vi "Destroy.vi"(8 "error in (no error)":errorcluster, 11 "Event Registration Refnum":refnum<event-registration>) -> (0 "error out":errorcluster)   [LabVIEW 2020, in "WebServiceImporter.lvlib" / "Main Panel.lvlib" / "Input WSDL.lvlib" / "Events.lvlib"]
uses:
  <vilib>/Platform/WebService/Main Panel/Pages/Input WSDL/Events/Events.lvlib
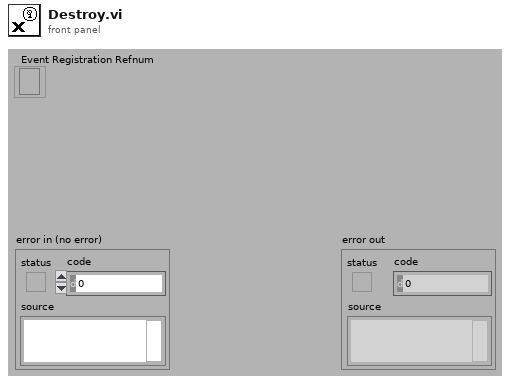
[diagram p1: front panel]
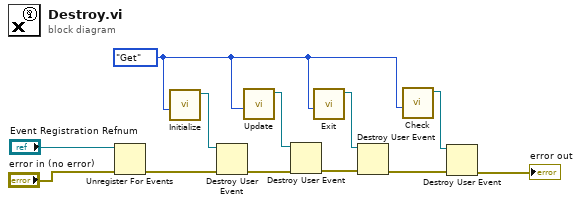
[diagram p0: block diagram]
diagram:
  w1 = enum16{"Get", "Set"}."Get" ("Operation")
  n1 = Unregister For Events(event registration refnum="Event Registration Refnum", error in="error in (no error)") -> (error out=w11:errorcluster)
  n2 = call <vilib>:"Initialize.vi"("Operation"=w1) -> ("user event (out)"=w10:refnum<user-event>)  [unwired: 10 in]
  n3 = Destroy User Event(user event=w10, error in=w11) -> (error out=w4:errorcluster)
  n4 = call <vilib>:"Update.vi"("Operation"=w1) -> ("user event (out)"=w2:refnum<user-event>)  [unwired: 9 in, 1 out]
  n5 = Destroy User Event(user event=w2, error in=w4) -> (error out=w3:errorcluster)
  n6 = call <vilib>:"Exit.vi"("Operation"=w1) -> ("user event (out)"=w9:refnum<user-event>)  [unwired: 9 in, 1 out]
  n7 = Destroy User Event(user event=w9, error in=w3) -> (error out=w8:errorcluster)
  n8 = call <vilib>:"Check.vi"("Operation"=w1) -> ("user event (out)"=w7:refnum<user-event>)  [unwired: 9 in, 1 out]
  n9 = Destroy User Event(user event=w7, error in=w8) -> (error out=→"error out":errorcluster)
